vi "FindAllActors.vi"(8 "error in (no error)":errorcluster, 11 "CS++MessageMakerMain in":refnum<class "CS++MessageMakerMain.lvclass">) -> (0 "error out":errorcluster, 3 "CS++MessageMakerMain out":refnum<class "CS++MessageMakerMain.lvclass">)   [LabVIEW 2015, in "CS++MessageMakerMain.lvlib" / "CS++MessageMakerMain.lvclass"]
doc: "Search for all Actors in a Project. Needed during the Initilaization procedure."
uses:
  CS++MessageMakerMain.lvclass
  CS++MessageMakerMain.lvclass/CS++MessageMakerMain.ctl
  CSPP_Actor/CS++Actor.lvclass
  CSPP_Actor/CS++Actor.lvclass/CS++Actor.ctl
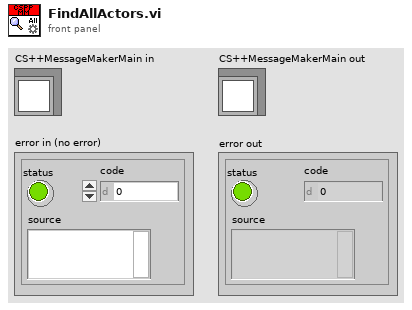
[diagram p1: front panel]
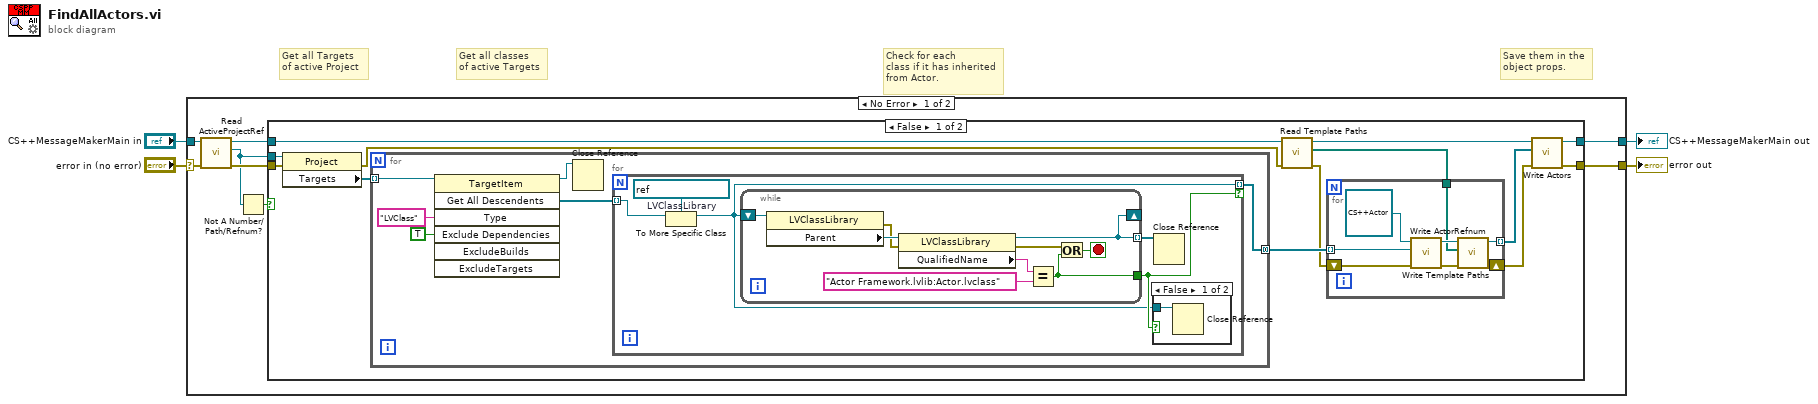
[diagram p0: block diagram]
diagram:
  # "Save them in the\nobject props."
  # "Check for each\nclass if it has inherited\nfrom Actor."
  # "Get all classes\nof active Targets"
  # "Get all Targets\nof active Project"
  n1 = case shown="No Error" "error in (no error)" {
    selector: "error in (no error)" -> [w11 w58]
    tunnel: [w9 w58] -> w3
    tunnel: [w8 w57] -> w1
    tunnel: "CS++MessageMakerMain in" -> [w12 w57]
    frame No Error {
      n2 = call "Read ActiveProjectRef.vi"("error in (no error)"=w11, "CS++MessageMakerMain in"=w12) -> ("error out"=w10:errorcluster, "ActiveProjectRef"=w6:refnum<vi>, "CS++MessageMakerMain out"=w7:refnum<class "CS++MessageMakerMain.lvclass">)  [unwired: 7 in]
      n3 = Not A Number/Path/Refnum?(number/path/refnum=w6) -> (NaN/Path/Refnum?=w5:bool)
      n4 = case shown="False" w5 {
        tunnel: w6 -> [w25 _]
        tunnel: w10 -> [w24 w55]
        tunnel: [w22 w55] -> w9
        tunnel: [w21 w56] -> w8
        tunnel: w7 -> [w15 w56]
        frame False {
          n5 = property class="Project"(reference=w25, error in=w24) -> (error out=w17:errorcluster, "Targets"=w23:refnum<vi>[])  [unwired: 1 out]
          n6 = for {
            tunnel: w23 -> [w38] mode=indexing
            tunnel: [w34] -> w20 mode=concatenating
            n7 = invoke class="TargetItem" method="Get All Descendents"(reference=w38, "Type"="LVClass", "Exclude Dependencies"=TRUE ("ExcludeDependencies")) -> (reference out=w35:refnum<vi>, "All Descendents"=w36:refnum<vi>[])  [unwired: 4 in, 5 out]
            n8 = Close Reference(reference=w35) -> ()  [unwired: 1 in, 1 out]
            n9 = for {
              tunnel: w36 -> [w43] mode=indexing
              tunnel: [w40] -> w34 mode=indexing if=w41
              w44 = refnum<vi> refnum  # LVClassLibrary
              n10 = To More Specific Class(target class=w44, reference=w43) -> (specific class reference=w40:refnum<vi>)  [unwired: 1 in, 1 out]
              n11 = while {
                shift-right: [w48] -> _
                shift-left: w40 -> [w54]
                tunnel: [w48] -> w42 mode=indexing
                tunnel: [w47] -> w41
                stop <- w49 stop-if-true
                n12 = property class="LVClassLibrary"(reference=w54) -> (error out=w46:errorcluster, "Parent"=w50:refnum<vi>)  [unwired: 1 in, 1 out]
                n13 = property class="LVClassLibrary"(reference=w50, error in=w46) -> (reference out=w48:refnum<vi>, error out=w51:errorcluster, "QualifiedName"=w53:string)
                n14 = Equal?(x=w53, y="Actor Framework.lvlib:Actor.lvclass") -> (x = y?=w47:bool)
                n15 = Or(x=w51, y=w47) -> (x .or. y?=w49:bool)
              }
              n16 = case shown="False" w41 {
                tunnel: w40 -> [w45 _]
                frame False {
                  n17 = Close Reference(reference=w45) -> ()  [unwired: 1 in, 1 out]
                }
                frame True {
                }
              }
              n18 = Close Reference(reference=w42) -> ()  [unwired: 1 in, 1 out]
            }
          }
          n19 = call "Read Template Paths.vi"("error in (no error)"=w17, "CS++MessageMakerMain in"=w15) -> ("error out"=w16:errorcluster, "Template Paths"=w13:path[], "CS++MessageMakerMain out"=w14:refnum<class "CS++MessageMakerMain.lvclass">)  [unwired: 7 in]
          n20 = for {
            shift-right: [w29] -> w19
            shift-left: w16 -> [w31]
            tunnel: w20 -> [w32] mode=indexing
            tunnel: [w27] -> w18 mode=indexing
            tunnel: w13 -> [w26]
            n21 = call "Write ActorRefnum.vi"("error in (no error)"=w31, "ActorRefnum"=w32, "CS++Actor in"=refnum<class "CS++Actor.lvclass"> refnum ("CS++Actor.lvlib:CS++Actor.lvclass")) -> ("error out"=w30:errorcluster, "CS++Actor out"=w28:refnum<class "CS++Actor.lvclass">)  [unwired: 7 in]
            n22 = call "Write Template Paths.vi"("error in (no error)"=w30, "Template Paths"=w26, "CS++Actor in"=w28) -> ("error out"=w29:errorcluster, "CS++Actor out"=w27:refnum<class "CS++Actor.lvclass">)  [unwired: 7 in]
          }
          n23 = call "Write Actors.vi"("error in (no error)"=w19, "Actors"=w18, "CS++MessageMakerMain in"=w14) -> ("error out"=w22:errorcluster, "CS++MessageMakerMain out"=w21:refnum<class "CS++MessageMakerMain.lvclass">)  [unwired: 7 in]
        }
        frame True {
        }
      }
    }
    frame Error {
    }
  }
  "error out" <- w3
  "CS++MessageMakerMain out" <- w1
